vi "Speech-SetVoiceAudioDev.vi"(5 "Voice":u16, 7 "Audio Device":u16, 8 "error in":errorcluster, 9 "Volume":i32=100, 10 "Rate":i32, 11 "speech_voice_refs":T1) -> (0 "error out":errorcluster, 3 "speech_voice_refs (out)":T1, 4 "Voice (out)":u16, 6 "AudioDevice (out)":u16)   [LabVIEW 8.6]
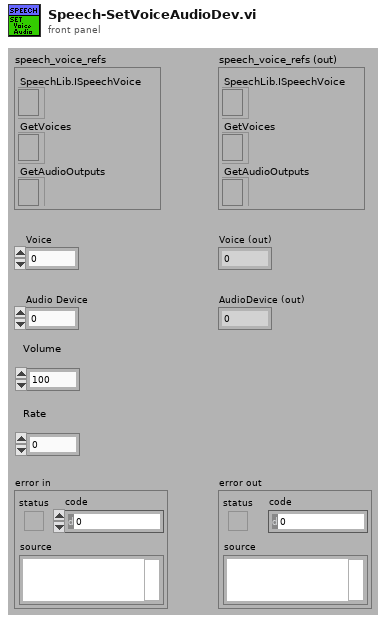
[diagram p1: front panel]
types:
  T1 = cluster{"SpeechLib.ISpeechVoice":refnum<k7>, "GetVoices":refnum<k7>, "GetAudioOutputs":refnum<k7>}
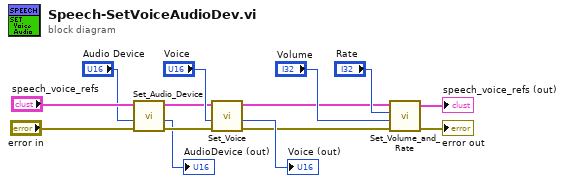
[diagram p0: block diagram]
diagram:
  n1 = call "Set_Audio_Device.vi"("error in (no error)"="error in", "AudioDevice"="Audio Device", "speech_voice_refs"="speech_voice_refs") -> ("error out"=w11:errorcluster, "AudioDevice (out)"=→"AudioDevice (out)":u16, "speech_voice_refs (out)"=w12:T1)  [unwired: 6 in]
  n2 = call "Set_Voice.vi"("error in (no error)"=w11, "Voice (in)"="Voice", "speech_voice_refs"=w12) -> ("error out"=w4:errorcluster, "Voice (out)"=→"Voice (out)":u16, "speech_voice_refs (out)"=w3:T1)  [unwired: 6 in]
  n3 = call "Set_Volume_and_Rate.vi"("error in (no error)"=w4, "Volume (100)"="Volume", "Speech Rate (0)"="Rate", "speech_voce_refs (in)"=w3) -> ("error out"=→"error out":errorcluster, "speech object references (out)"=→"speech_voice_refs (out)":T1)  [unwired: 6 in]
